vi "Close.vi"(8 "Error In":errorcluster, 10 "Enable Calendar Tree":bool=TRUE, 11 "Log In":refnum<file>) -> (0 "Error Out":errorcluster, 3 "Base Log Folder":path)   [LabVIEW 2017, in "Toolkit.lvlib" / "File.lvlib"]
uses:
  File.lvlib
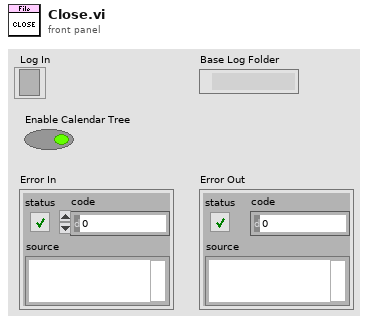
[diagram p1: front panel]
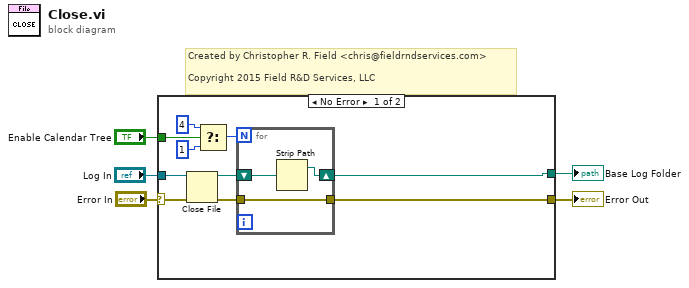
[diagram p0: block diagram]
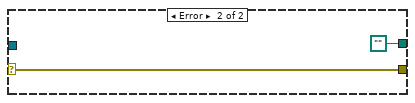
[diagram p2: hidden frame]
diagram:
  # "Created by Christopher R. Field <chris@fieldrndservices.com>\n\nCopyright 2015 Field R&D Services, LLC"
  n1 = case shown="No Error" "Error In" {
    selector: "Error In" -> [w14 w20]
    tunnel: "Log In" -> [w15 _]
    tunnel: [w11 path ""] -> w3
    tunnel: [w10 w20] -> w2
    tunnel: "Enable Calendar Tree" -> [w9 _]
    frame No Error {
      n2 = Close File(refnum=w15, error in=w14) -> (path=w13:path, error out=w12:errorcluster)
      n3 = Select(t=4, s=w9, f=1) -> (s? t:f=w7:i32)
      n4 = for {
        N: w7 -> [_]
        shift-right: [w17] -> w11
        shift-left: w13 -> [w18]
        tunnel: w12 -> [w16]
        tunnel: [w16] -> w10
        n5 = Strip Path(path=w18) -> (stripped path=w17:path)  [unwired: 1 out]
      }
    }
    frame Error {
    }
  }
  "Base Log Folder" <- w3
  "Error Out" <- w2
